vi "Get Control Reference by Label.vi"(8 "error in (no error)":errorcluster, 10 "Control Name":string, 11 "Control Refs":refnum<vi>[](array[refnum])) -> (0 "error out":errorcluster, 2 "Found?":bool, 3 "Control Ref":refnum<vi>)   [LabVIEW 2020, in "MacroAssert.lvlib"]
uses:
  MacroAssert.lvlib
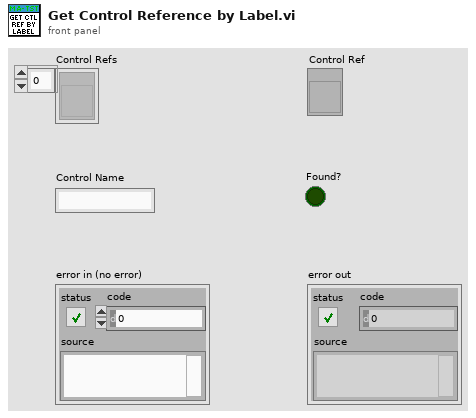
[diagram p1: front panel]
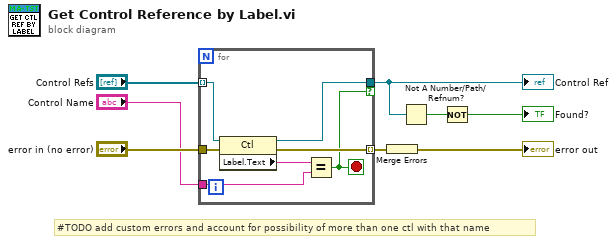
[diagram p0: block diagram]
diagram:
  # "#TODO add custom errors and account for possibility of more than one ctl with that name"
  n1 = for {
    tunnel: "Control Refs" -> [w15] mode=indexing
    tunnel: [w14] -> w3 if=w9
    tunnel: "Control Name" -> [w12]
    tunnel: [w11] -> w7 mode=indexing
    tunnel: "error in (no error)" -> [w10]
    stop <- w9 stop-if-true
    n2 = property class="Ctl"(reference=w15, error in=w10) -> (reference out=w14:refnum<vi>, error out=w11:errorcluster, "Label.Text"=w13:string)
    n3 = Equal?(x=w13, y=w12) -> (x = y?=w9:bool)
  }
  "Control Ref" <- w3
  n4 = Merge Errors(w7) -> (→"error out":errorcluster)
  n5 = Not A Number/Path/Refnum?(number/path/refnum=w3) -> (NaN/Path/Refnum?=w2:bool)
  n6 = Not(x=w2) -> (.not. x?=→"Found?":bool)
